vi "PrepareHWI.vi"(8 "error in (no error)":errorcluster, 9 "Master Device in":refnum<class "Master Device.lvclass">, 10 "Current Variables":T1[](array[typedef]), 11 "Slave_Line in":refnum<class "Slave_Line.lvclass">) -> (0 "error out":errorcluster, 2 "Master Device out":refnum<class "Master Device.lvclass">, 3 "Slave_Line out":refnum<class "Slave_Line.lvclass">)   [LabVIEW 2013, in "Slave_Line.lvclass"]
doc: "Prepare HWI will parse string table values to generate a hardware image for each device. Both variables and user functions can be pre-registered! This makes setting variables optional."
uses:
  Slave_Line.lvclass
  Master Device/Master Device.lvclass
  TypeDefs/Active procedure variables.ctl
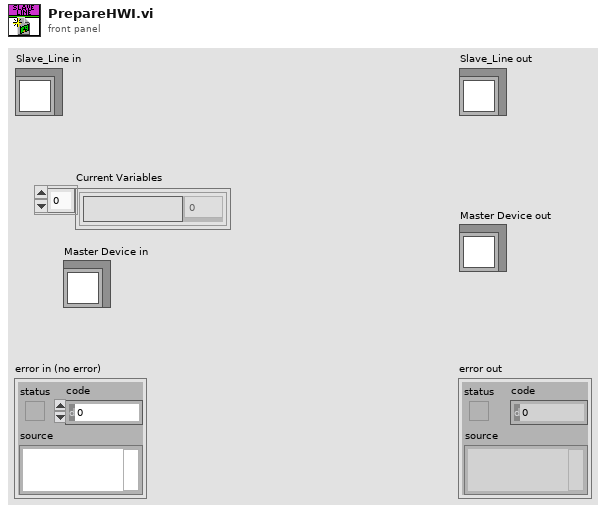
[diagram p1: front panel]
types:
  T1 = typedef "Active procedure variables.ctl" = cluster{"Procedure variable":string, "Value":dbl}
  T2 = typedef "SlaveInfo.ctl" = cluster{"Triggering":bool[][], "Ramp Info":T3[], "Line Inversion":bool[], "Slaved Digital Channels":cluster{"Master Channel Number":i32, "Output States":bool[]}[]}
  T3 = typedef "RampInfo.ctl" = cluster{"Table Ramp Index":i32, "Ramp Time":dbl, "Number of Steps":i32, "Instruction Array Index":i32}
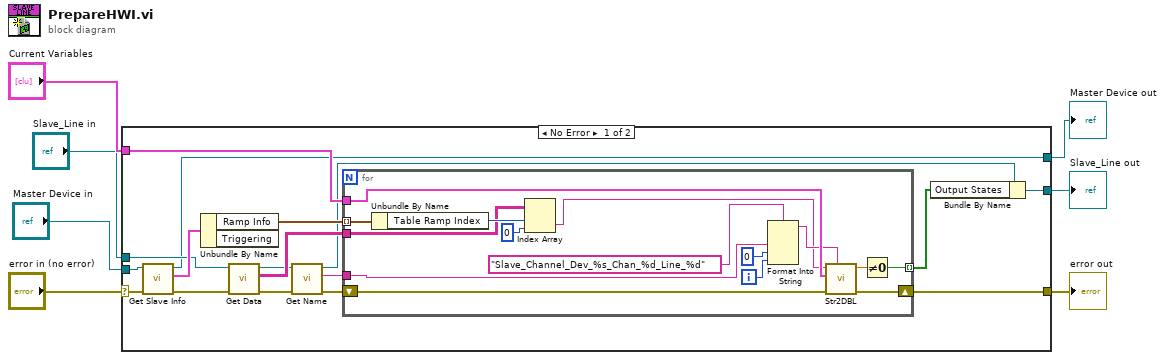
[diagram p0: block diagram]
diagram:
  n1 = case shown="No Error" "error in (no error)" {
    selector: "error in (no error)" -> [w19 w42]
    tunnel: "Current Variables" -> [w21 _]
    tunnel: "Master Device in" -> [w20 w41]
    tunnel: "Slave_Line in" -> [w14 w40]
    tunnel: [w12 w42] -> w3
    tunnel: [w11 w41] -> w2
    tunnel: [w10 w40] -> w1
    frame No Error {
      n2 = call-dynamic "Get Slave Info.vi"("error in (no error)"=w19, "Master Device in"=w20) -> ("error out"=w15:errorcluster, "Slave Info"=w18:T2, "Master Device out"=w11:refnum<class "Master Device.lvclass">)  [unwired: 7 in]
      n3 = Unbundle By Name(w18) -> ("Ramp Info"=w23:T3[])  [unwired: 1 out]
      n4 = call-dynamic "Get Data.vi"("error in (no error)"=w15, "Device in"=w14) -> ("error out"=w24:errorcluster, "Table Indicator"=w22:string[][], "Device out"=w13:refnum<class "Slave_Line.lvclass">)  [unwired: 6 in]
      n5 = call-dynamic "Get Name.vi"("error in (no error)"=w24, "Device in"=w13) -> ("error out"=w16:errorcluster, "Name"=w17:string, "Device out"=w9:refnum<class "Slave_Line.lvclass">)  [unwired: 7 in]
      n6 = for {
        tunnel: w23 -> [w39] mode=indexing
        tunnel: w22 -> [w37]
        tunnel: w17 -> [w35]
        tunnel: w21 -> [w33]
        shift-right: [w31] -> w12
        shift-left: w16 -> [w32]
        tunnel: [w30] -> w8 mode=indexing
        i -> [w34]
        n7 = Unbundle By Name(w39) -> ("Table Ramp Index"=w38:i32)
        n8 = Index Array(array=w37, index (row)=w38, index (col)=0 ("disabled index (col)")) -> (element=w25:string)
        n9 = Format Into String(format string="Slave_Channel_Dev_%s_Chan_%d_Line_%d", w35, 0 ("input 2"), w34) -> (resulting string=w29:string)  [unwired: 2 in, 1 out]
        n10 = call "Str2DBL.vi"("Error Locator"=w29, "error in (no error)"=w32, "Current Variable settings"=w33, "formula"=w25) -> ("error out"=w31:errorcluster, "y value"=w28:dbl)  [unwired: 4 in]
        n11 = Not Equal To 0?(x=w28) -> (x != 0?=w30:bool)
      }
      n12 = Bundle By Name(cluster=w9, "Output States"=w8) -> (w10:refnum<class "Slave_Line.lvclass">)
    }
    frame Error {
    }
  }
  "error out" <- w3
  "Slave_Line out" <- w1
  "Master Device out" <- w2
